vi "Read Magnetometer.vi"(8 "error in (no error)":errorcluster, 11 "LSM9DS1 IMU in":refnum<class "LSM9DS1 IMU.lvclass">) -> (0 "error out":errorcluster, 2 "Magnetometer Values (gauss)":T1, 3 "LSM9DS1 IMU out":refnum<class "LSM9DS1 IMU.lvclass">)   [LabVIEW 2020, in "LSM9DS1 IMU.lvclass"]
doc: "Read 3-axis magnetometer data in units of Gauss."
uses:
  LSM9DS1 IMU.lvclass
  3 Axis Values.ctl
  LSM9DS1 IMU.lvclass/LSM9DS1 IMU.ctl
  Read Magnetometer I2C.vi
  Write Magnetometer I2C.vi
  Read Magnetometer Range.vi
  LINX I2C/LINX I2C.lvclass
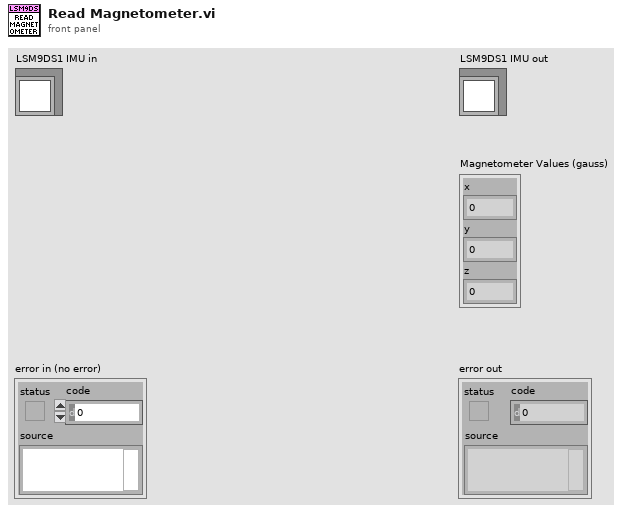
[diagram p1: front panel]
types:
  T1 = typedef "LSM9DS1 IMU.lvclass/3 Axis Values.ctl" = cluster{"x":dbl, "y":dbl, "z":dbl}
  T2 = typedef "LSM9DS1 IMU.lvclass/Magnetometer Range.ctl" = enum16{"4 gauss", "8 gauss", "12 gauss", "16 gauss"}
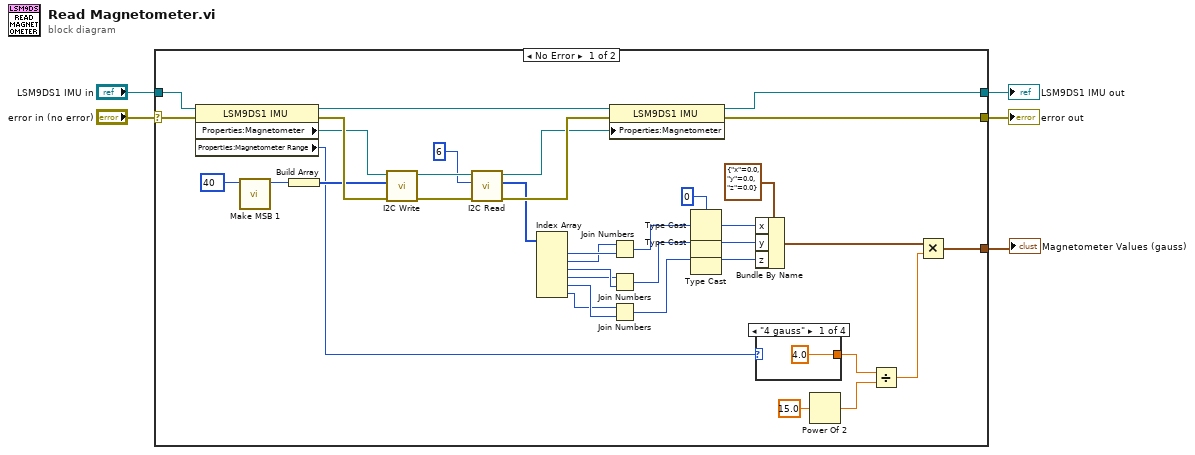
[diagram p0: block diagram]
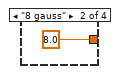
[diagram p2: hidden frame]
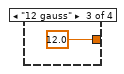
[diagram p3: hidden frame]
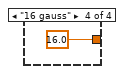
[diagram p4: hidden frame]
diagram:
  n1 = case shown="No Error" "error in (no error)" {
    selector: "error in (no error)" -> [w32 w48]
    tunnel: [w33 w48] -> w4
    tunnel: [w37 w47] -> w2
    tunnel: "LSM9DS1 IMU in" -> [w42 w47]
    tunnel: [w6 _] -> w1
    frame No Error {
      w13 = i16 0
      n2 = property class="LSM9DS1 IMU"(reference=w42, error in=w32) -> (reference out=w38:refnum<class "LSM9DS1 IMU.lvclass">, error out=w36:errorcluster, "Properties:Magnetometer"=w31:refnum<class "LINX I2C.lvclass">, "Properties:Magnetometer Range"=w8:T2)
      n3 = call "Make MSB 1.vi"("Register Address"=u8 40) -> ("Register Address | 0x80"=w21:u8)  [unwired: 10 in]
      n4 = Build Array(w21) -> (w20:u8[])
      n5 = call "I2C Write.vi"("error in (no error)"=w36, "Bytes to Write"=w20, "LINX I2C in"=w31) -> ("error out"=w41:errorcluster, "LINX I2C out"=w40:refnum<class "LINX I2C.lvclass">)  [unwired: 7 in]
      n6 = call-dynamic "I2C Read.vi"("error in (no error)"=w41, "# Bytes to Read"=u8 6, "LINX I2C in"=w40) -> ("error out"=w35:errorcluster, "Bytes Read"=w29:u8[], "LINX I2C out"=w30:refnum<class "LINX I2C.lvclass">)  [unwired: 6 in]
      n7 = Index Array(array=w29) -> (element #1=w28:u8, element #2=w27:u8, element #3=w26:u8, element #4=w25:u8, element #5=w24:u8, element #6=w23:u8)  [unwired: 6 in]
      n8 = property class="LSM9DS1 IMU"(reference=w38, error in=w35, "Properties:Magnetometer"=w30) -> (reference out=w37:refnum<class "LSM9DS1 IMU.lvclass">, error out=w33:errorcluster)
      n9 = Join Numbers(hi=w27, lo=w28) -> ((hi.lo)=w19:u16)
      n10 = Join Numbers(hi=w25, lo=w26) -> ((hi.lo)=w18:u16)
      n11 = Join Numbers(hi=w23, lo=w24) -> ((hi.lo)=w17:u16)
      n12 = Type Cast(type=w13, x=w19) -> (*(type *) &x=w16:i16)
      n13 = Type Cast(type=w13, x=w18) -> (*(type *) &x=w15:i16)
      n14 = Type Cast(type=w13, x=w17) -> (*(type *) &x=w14:i16)
      n15 = Bundle By Name(cluster=T1 {"x"=0.0, "y"=0.0, "z"=0.0} ("Gyro Values"), "x"=w16, "y"=w15, "z"=w14) -> (w7:T1)
      n16 = case shown="\"4 gauss\"" w8 {
        tunnel: [4.0 8.0 12.0 16.0] -> w10
        frame "4 gauss" {
        }
        frame "8 gauss" {
        }
        frame "12 gauss" {
        }
        frame "16 gauss" {
        }
      }
      n17 = Power Of 2(x=15.0) -> (2^x=w11:dbl)
      n18 = Divide(x=w10, y=w11) -> (x/y=w9:dbl)
      n19 = Multiply(x=w7, y=w9) -> (x*y=w6:T1)
    }
    frame Error {
    }
  }
  "error out" <- w4
  "LSM9DS1 IMU out" <- w2
  "Magnetometer Values (gauss)" <- w1
